vi "TDK-Lambda Z Set and Read Output Parameters by Event.vi"() -> ()   [LabVIEW 2013]
doc: "This example shows how to configure output and take readings.\n\n<b>Note:</b>\n1. Set Property Communication Parameters\n2. Set Required Output Values and then RUN"
uses:
  TDK-Lambda Z.lvlib
panel:
  in  "Configuration":T1={"Address"=6, "Baud Rate"=9600, "Language Selector"=1} {"Language Selector" items=["GEN", "SCPI"]; "Baud Rate" items=["1200"=1200, "2400"=2400, "4800"=4800, "9600"=9600, "19200"=19200, "38400"=38400, "57600"=57600, "115200"=115200]}
  out "Output Power (W)":dbl format="%.4f"
  out "Output Current (A)":dbl format="%.4f"
  out "Output Voltage (V)":dbl format="%.4f"
  in  "Current Limit (0A)":dbl format="%.4f"
  in  "Voltage Limit (0V)":dbl format="%.4f"
  in  "Output (F: Off)":bool
  in  "VISA resource name":refnum<visa-resource-name>
  in  "Reset(True)":bool
  in  "STOP":bool
  # "(c) 2014-2015 TDK-Lambda.  ALL RIGHTS RESERVED."
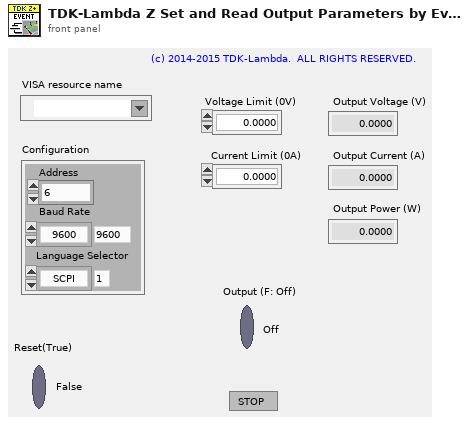
[diagram p1: front panel]
types:
  T1 = cluster{"Address":i16, "Baud Rate":u32, "Language Selector":i16}
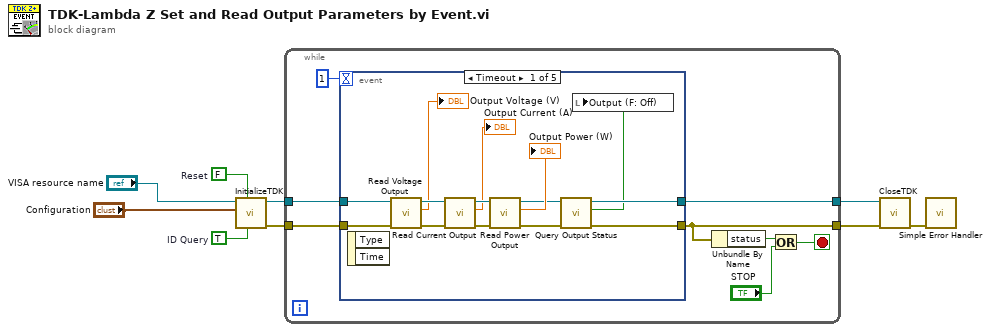
[diagram p0: block diagram]
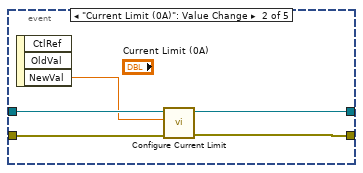
[diagram p2: hidden frame]
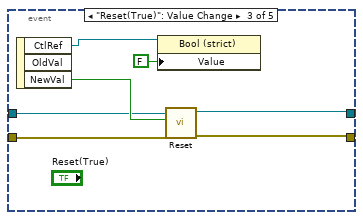
[diagram p3: hidden frame]
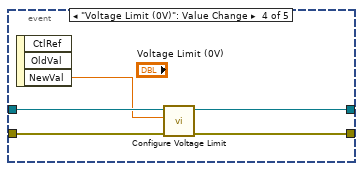
[diagram p4: hidden frame]
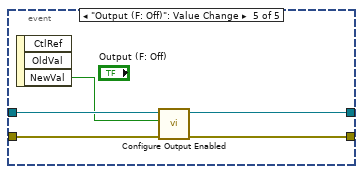
[diagram p5: hidden frame]
diagram:
  w2 = TRUE  # ID Query
  w3 = FALSE  # Reset
  n1 = call "InitializeTDK.vi"("ID Query (True)"=w2, "Reset(True)"=w3, "Configuration"="Configuration", "VISA resource name"="VISA resource name") -> ("error out"=w7:errorcluster, "VISA resource name out"=w6:refnum<visa-resource-name>)  [unwired: 6 in]
  n2 = while {
    tunnel: w6 -> [w17]
    tunnel: [w11] -> w9
    tunnel: w7 -> [w16]
    tunnel: [w10] -> w8
    stop <- w14 stop-if-true
    n3 = event shown="[0] Timeout" {
      selector: _ -> [_ _ _ _ _]
      dyn-events: _ -> [_ _ _ _ _]
      timeout: 1 -> [_ _ _ _ _]
      tunnel: w17 -> [w31 w36 w40 w48 w53]
      tunnel: [w20 w34 w39 w46 w50] -> w11
      tunnel: w16 -> [w28 w35 w43 w47 w52]
      tunnel: [w19 w33 w42 w45 w51] -> w10
      event Timeout {
        n4 = event-data() -> ()  [unwired: 1 in, 2 out]
        n5 = call "Read Voltage Output .vi"("error in (no error)"=w28, "VISA resource name"=w31) -> ("error out"=w24:errorcluster, "Output Voltage (V)"=→"Output Voltage (V)":dbl, "VISA resource name out"=w30:refnum<visa-resource-name>)  [unwired: 7 in]
        n6 = call "Read Current Output.vi"("error in (no error)"=w24, "VISA resource name"=w30) -> ("error out"=w27:errorcluster, "Output Current (A)"=→"Output Current (A)":dbl, "VISA resource name out"=w29:refnum<visa-resource-name>)  [unwired: 7 in]
        n7 = call "Read Power Output.vi"("error in (no error)"=w27, "VISA resource name"=w29) -> ("error out"=w22:errorcluster, "Output Power (W)"=→"Output Power (W)":dbl, "VISA resource name out"=w21:refnum<visa-resource-name>)  [unwired: 7 in]
        n8 = call "Query Output Status.vi"("error in (no error)"=w22, "VISA resource name"=w21) -> ("error out"=w19:errorcluster, "Output On"=w18:bool, "VISA resource name out"=w20:refnum<visa-resource-name>)  [unwired: 7 in]
        n9 = local write "Output (F: Off)"(w18) -> ()
      }
      event "Current Limit (0A)": Value Change {
        n10 = event-data() -> ("NewVal"=w32:dbl)  [unwired: 1 in, 2 out]
        n11 = call "Configure Current Limit.vi"("error in (no error)"=w35, "Current Limit (0A)"=w32, "VISA resource name"=w36) -> ("error out"=w33:errorcluster, "VISA resource name out"=w34:refnum<visa-resource-name>)  [unwired: 7 in]
      }
      event "Reset(True)": Value Change {
        n12 = event-data() -> ("CtlRef"=w38:refnum<vi>, "NewVal"=w41:bool)  [unwired: 1 in, 1 out]
        n13 = property class="Bool (strict)"(reference=w38, "Value"=FALSE) -> ()  [unwired: 1 in, 2 out]
        n14 = call "Reset.vi"("error in (no error)"=w43, "Reset (False: Off)"=w41, "VISA resource name"=w40) -> ("error out"=w42:errorcluster, "VISA resource name out"=w39:refnum<visa-resource-name>)  [unwired: 7 in]
      }
      event "Voltage Limit (0V)": Value Change {
        n15 = event-data() -> ("NewVal"=w44:dbl)  [unwired: 1 in, 2 out]
        n16 = call "Configure Voltage Limit.vi"("error in (no error)"=w47, "Voltage Limit (0V)"=w44, "VISA resource name"=w48) -> ("error out"=w45:errorcluster, "VISA resource name out"=w46:refnum<visa-resource-name>)  [unwired: 7 in]
      }
      event "Output (F: Off)": Value Change {
        n17 = event-data() -> ("NewVal"=w49:bool)  [unwired: 1 in, 2 out]
        n18 = call "Configure Output Enabled.vi"("error in (no error)"=w52, "Enable Output (F: Off)"=w49, "VISA resource name"=w53) -> ("error out"=w51:errorcluster, "VISA resource name out"=w50:refnum<visa-resource-name>)  [unwired: 7 in]
      }
    }
    n19 = Unbundle By Name(w10) -> ("status"=w13:bool)
    n20 = Or(x=w13, y="STOP") -> (x .or. y?=w14:bool)
  }
  n21 = call "CloseTDK.vi"("error in (no error)"=w8, "VISA resource name"=w9) -> ("error out"=w4:errorcluster)  [unwired: 9 in]
  n22 = call <vilib>:"Simple Error Handler.vi"("error in (no error)"=w4) -> ()  [unwired: 4 in, 5 out]
